vi "Read Chunked Body.vi"(8 "error in (no error)":errorcluster, 10 "Max Size (50MB)":u64=52428800, 11 "Stream in":refnum<k5>) -> (0 "error out":errorcluster, 2 "Body":string, 3 "Stream out":refnum<k5>)   [LabVIEW 2020, in "HTTP Utils.lvlib" / "Request.lvclass"]
uses:
  Request.lvclass
  Request.lvclass/Request.ctl
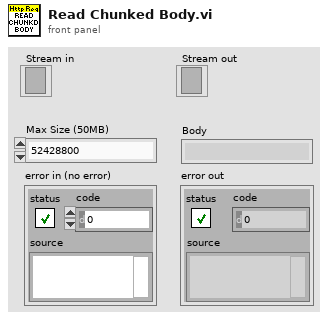
[diagram p1: front panel]
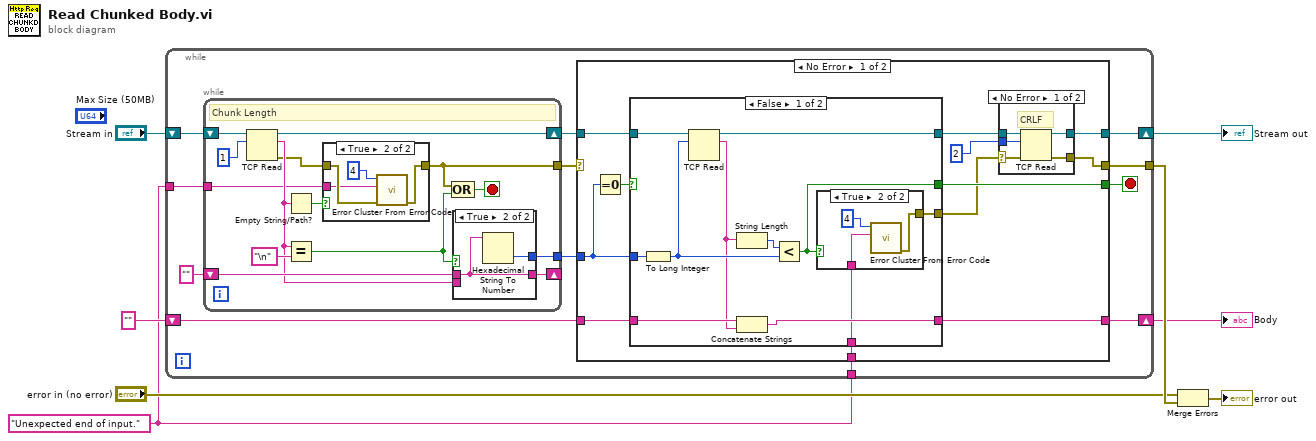
[diagram p0: block diagram]
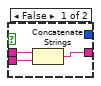
[diagram p3: hidden frame]
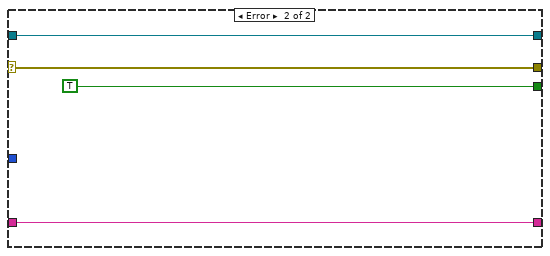
[diagram p7: hidden frame]
diagram:
  w1 = "Unexpected end of input."
  n1 = while {
    shift-right: [w11] -> w5
    shift-left: "Stream in" -> [w20]
    shift-right: [w12] -> w3
    shift-left: "" -> [w15]
    tunnel: [w14] -> w8
    tunnel: w1 -> [w10]
    tunnel: w1 -> [w9]
    stop <- w13 stop-if-true
    n2 = while {
      shift-right: [w32] -> w18
      shift-left: w20 -> [w34]
      shift-right: [w27] -> _
      shift-left: "" -> [w28]
      tunnel: [w21] -> w17
      tunnel: [w26] -> w16
      tunnel: w10 -> [w22]
      stop <- w30 stop-if-true
      # "Chunk Length"
      n3 = TCP Read(connection ID=w34, bytes to read=1 ("Count")) -> (connection ID out=w32:refnum<k5>, data out=w25:string, error out=w24:errorcluster)  [unwired: 3 in]
      n4 = Empty String/Path?(string/path=w25) -> (empty?=w23:bool)
      n5 = Equal?(x=w25, y="\n") -> (x = y?=w29:bool)
      n6 = case shown="True" w23 {
        tunnel: w24 -> [w35 w37]
        tunnel: [w35 w39] -> w21
        tunnel: w22 -> [_ w36]
        frame False {
        }
        frame True {
          n7 = call <vilib>:"Error Cluster From Error Code.vi"("error in (no error)"=w37, "error message (\"\")"=w36, "error code (0)"=4) -> ("error out"=w39:errorcluster)  [unwired: 6 in]
        }
      }
      n8 = Compound Arithmetic op=OR(w21, w29) -> (w30:bool)
      n9 = case shown="True" w29 {
        tunnel: w28 -> [w42 w44]
        tunnel: w25 -> [w41 _]
        tunnel: [w40 w44] -> w27
        tunnel: [_ w43] -> w26
        frame False {
          n10 = Concatenate Strings(w42, w41) -> (w40:string)
        }
        frame True {
          n11 = Hexadecimal String To Number(string=w44) -> (number=w43:u32)  [unwired: 2 in, 1 out]
        }
      }
    }
    n12 = case shown="No Error" w17 {
      selector: w17 -> [_ w84]
      tunnel: w18 -> [w56 w81]
      tunnel: w16 -> [w51 _]
      tunnel: w15 -> [w53 w82]
      tunnel: [w49 w84] -> w14
      tunnel: [w47 TRUE] -> w13
      tunnel: [w52 w82] -> w12
      tunnel: [w50 w81] -> w11
      tunnel: w9 -> [w46 _]
      frame No Error {
        n13 = Equal To 0?(x=w51) -> (x = 0?=w48:bool)
        n14 = case shown="False" w48 {
          selector: w48 -> [_ w78]
          tunnel: w56 -> [w74 w80]
          tunnel: [w73 w80] -> w55
          tunnel: w53 -> [w72 w79]
          tunnel: [w71 w79] -> w52
          tunnel: w51 -> [w70 _]
          tunnel: [w64 w78] -> w47
          tunnel: w46 -> [w66 _]
          tunnel: [w65 _] -> w45
          frame False {
            n15 = To Long Integer(number=w70) -> (32bit integer=w68:i32)
            n16 = TCP Read(connection ID=w74, bytes to read=w68) -> (connection ID out=w73:refnum<k5>, data out=w67:string)  [unwired: 3 in, 1 out]
            n17 = String Length(string=w67) -> (length=w69:i32)
            n18 = Concatenate Strings(w72, w67) -> (w71:string)
            n19 = Less?(x=w69, y=w68) -> (x < y?=w64:bool)
            n20 = case shown="True" w64 {
              tunnel: [_ w77] -> w65
              tunnel: w66 -> [_ w75]
              frame False {
              }
              frame True {
                n21 = call <vilib>:"Error Cluster From Error Code.vi"("error message (\"\")"=w75, "error code (0)"=4) -> ("error out"=w77:errorcluster)  [unwired: 7 in]
              }
            }
          }
          frame True {
          }
        }
        n22 = case shown="No Error" w45 {
          selector: w45 -> [w57 w63]
          tunnel: w55 -> [w61 w62]
          tunnel: 2 ("Count") -> [w60 _]
          tunnel: [w59 w62] -> w50
          tunnel: [w58 w63] -> w49
          frame No Error {
            # "CRLF"
            n23 = TCP Read(connection ID=w61, bytes to read=w60, error in (no error)=w57) -> (connection ID out=w59:refnum<k5>, error out=w58:errorcluster)  [unwired: 2 in, 1 out]
          }
          frame Error {
          }
        }
      }
      frame Error {
      }
    }
  }
  "Stream out" <- w5
  "Body" <- w3
  n24 = Merge Errors("error in (no error)", w8) -> (→"error out":errorcluster)
